vi "2 PureWindHeadingGoodness.vi"(4 "Heading to Test":dbl) -> (1 "Goodness":dbl)   [LabVIEW 2011]
doc: "Takes the absolute wind vector, the heading of your next waypoint, and a test heading and outputs a goodness value for the test heading. The criteria is the speed to get to the waypoint.\n\nThe goodness is evaluated by taking the softmax of an angle with all possible complimenting angles (i.e. if the test heading is 10 degrees it is matched with -1 through -89; note that angles are adjusted to be degrees from directly at the waypoint). The specific calculation for finding the net velocity of a pair of angles requires the velocities from the polar plot."
uses:
  2 Globals/2 Global.vi
panel:
  # "Inputs"
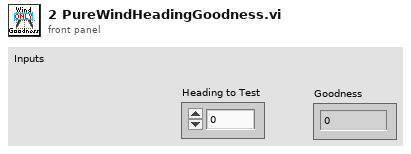
[diagram p1: front panel]
types:
  T1 = typedef "apparent wind.ctl" = cluster{"Toward Fore":dbl, "Toward Starboard":dbl}
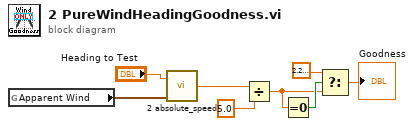
[diagram p0: block diagram]
diagram:
  n1 = global read "2 Global.vi" "Apparent Wind"() -> (w3:T1)
  n2 = call "2 absolute_speed.vi"("Wind Vector"=w3, "Boat Angle"="Heading to Test") -> ("Velocity"=w1:dbl)
  n3 = Divide(x=w1, y=5.0) -> (x/y=w4:dbl)
  n4 = Equal To 0?(x=w4) -> (x = 0?=w6:bool)
  n5 = Select(t=2.220446049250313e-16, s=w6, f=w4) -> (s? t:f=→"Goodness":dbl)
